vi "Controllers.vi"() -> ()   [LabVIEW 2018]
uses:
  Classes/Controller/I-O/I-O.lvclass
  C:/Program Files (x86)/Aerotech/A3200/LabVIEW/2010/Bin/Aerotech.A3200.dll
  Program Files (x86)/Aerotech/A3200/LabVIEW/2010/Bin/Aerotech.A3200.dll
  Classes/Controller/Controllers.ctl
  Classes/Controller/Controller.lvclass
panel:
  in  "Cluster":T1={"I-O.lvclass"=refnum, "Gantry"=refnum, "Dispenser"="COM1"}
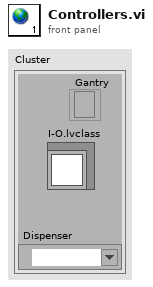
[diagram p1: front panel]
types:
  T1 = typedef "Controller.lvclass/Controllers.ctl" = cluster{"I-O.lvclass":refnum<class "I-O.lvclass">, "Gantry":refnum<k24>, "Dispenser":refnum<visa-resource-name>}
diagram:
